vi "WriteDAC_1212(Host).vi"(0 "FPGA Interface In":refnum<k20>, 1 "Selected DAC":u8(ring)=20 items=["DAC0 (A)", "DAC1 (B)"], 2 "Address":u8 max=31 format="%.0x", 3 "error in (no error)":errorcluster, 4 "Data":u8 max=31 format="%.0x") -> (5 "FPGA Interface Out":refnum<k20>, 7 "error out":errorcluster)   [LabVIEW 2018]
uses:
  <vilib>/Utility/error.llb/Error Cluster From Error Code.vi
  <vilib>/rvi/errors/niLvFpgaAdjustHostInterfaceError.vi
  <vilib>/rvi/interface/nirviReadWriteControl/nirviReadWriteControl.xnode
  NiFpgaLv.dll
  <vilib>/rvi/interface/Simulation/niFpgaSimulationCallBeginRW.vi
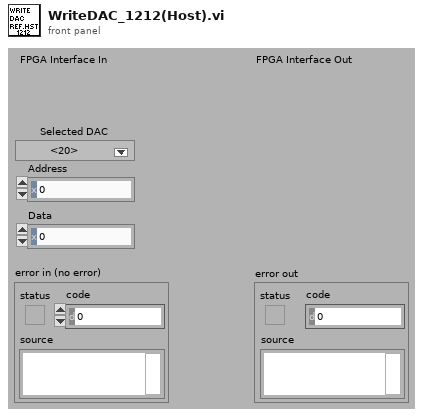
[diagram p1: front panel]
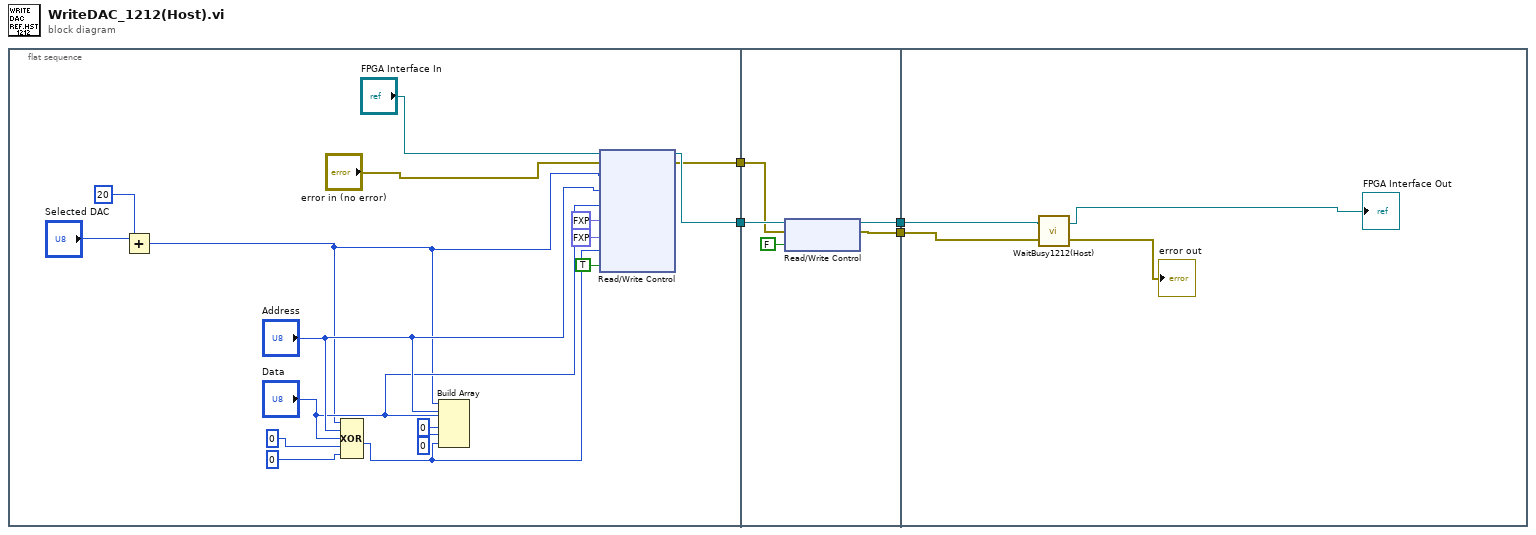
[diagram p0: block diagram]
diagram:
  n1 = flat-sequence {
    tunnel: [w8] -> w4
    tunnel: [w7] -> w3
    tunnel: w4 -> [w26]
    tunnel: w3 -> [w25]
    tunnel: [w23] -> w2
    tunnel: [w22] -> w1
    tunnel: w2 -> [w30]
    tunnel: w1 -> [w29]
    frame #0 {
      n2 = Add(x="Selected DAC", y=u8 20) -> (x+y=w6:u8)
      n3 = Compound Arithmetic op=XOR(w6, "Address", "Data", u8 0, u8 0) -> (w11:u8)
      n4 = Build Array(w6, "Address", "Data", u8 0 ("element"), u8 0 ("element"), w11) -> ()  [unwired: 1 out]
      n5 = xnode "Read/Write Control"("FPGA VI Reference In"="FPGA Interface In", "error in"="error in (no error)", "DataI2c0"=w6, "DataI2c1"="Address", "DataI2c2"="Data", "DataI2c3"=fxp<+,8,8> 0.0 ("IO Module\\datai2c3"), "DataI2c4"=fxp<+,8,8> 0.0 ("IO Module\\datai2c4"), "DataI2c5"=w11, "StartWRI2c"=TRUE ("IO Module\\starwri2c")) -> ("FPGA VI Reference Out"=w8:refnum<k20>, "error out"=w7:errorcluster)
    }
    frame #1 {
      n6 = xnode "Read/Write Control"("FPGA VI Reference In"=w26, "error in"=w25, "StartWRI2c"=FALSE) -> ("FPGA VI Reference Out"=w23:refnum<k20>, "error out"=w22:errorcluster)
    }
    frame #2 {
      n7 = call "WaitBusy1212(Host).vi"("error in"=w29, "FPGA VI Reference In"=w30) -> ("error out"=→"error out":errorcluster, "FPGA VI Reference Out"=→"FPGA Interface Out":refnum<k20>)
    }
  }
